vi "TTL high.vi"(1 "Line":i32, 2 "Port":i32, 3 "Do this?":bool=TRUE, 4 "Input":i64[][](array[numeric])=[[-64400000, 1, 6, 0], [-64399000, 0, 12, 0], [-64398000, 0, 12, 1], [-900000, 1, 9, 1], [0, 0, 4, 0], [0, 0, 9, 1], [0, 0, 15, 1], [0, 1, 0, 1], [0, 1, 1, 1], [0, 1, 2, 0], [0, 1, 3, 0], [0, 1, 4, 0], [0, 1, 5, 1], [0, 1, 12, 1], [1000, 1, 7, 0], [10000, 0, 2, 0], [495000, 0, 10, 1], [499000, 0, 6, 0], [501000, 0, 6, 1], [520000, 0, 10, 0], [869000, 0, 11, 1], [896000, 0, 2, 0], [896500, 0, 3, 1], [896500, 0, 9, 0], [896500, 0, 13, 0], [897000, 0, 5, 0], [897000, 1, 7, 1], [898740, 1, 12, 0], [899000, 0, 1, 1], [899000, 0, 4, 0], [899000, 0, 11, 0], [899000, 1, 1, 0], [899000, 1, 13, 1], [899200, 0, 14, 0], [899350, 0, 2, 0], [899400, 0, 14, 1], [899500, 0, 1, 0], [899500, 0, 2, 0], [899500, 0, 4, 0], [900000, 0, 2, 0], [900000, 0, 13, 0], [900000, 1, 1, 1], [900000, 1, 4, 1], [900000, 1, 5, 0], [900000, 1, 7, 0], [900000, 1, 12, 1], [901000, 0, 3, 0], [904000, 0, 5, 0], [904000, 1, 13, 0]], 5 "Absolute start time (ms)":dbl=1400.0 format="%.3f") -> (0 "Output":i64[][](array[numeric])=[[-64400000, 1, 6, 0], [-64399000, 0, 12, 0], [-64398000, 0, 12, 1], [-900000, 1, 9, 1], [0, 0, 4, 0], [0, 0, 9, 1], [0, 0, 15, 1], [0, 1, 0, 1], [0, 1, 1, 1], [0, 1, 2, 0], [0, 1, 3, 0], [0, 1, 4, 0], [0, 1, 5, 1], [0, 1, 12, 1], [1000, 1, 7, 0], [10000, 0, 2, 0], [495000, 0, 10, 1], [499000, 0, 6, 0], [501000, 0, 6, 1], [520000, 0, 10, 0], [869000, 0, 11, 1], [896000, 0, 2, 0], [896500, 0, 3, 1], [896500, 0, 9, 0], [896500, 0, 13, 0], [897000, 0, 5, 0], [897000, 1, 7, 1], [898740, 1, 12, 0], [899000, 0, 1, 1], [899000, 0, 4, 0], [899000, 0, 11, 0], [899000, 1, 1, 0], [899000, 1, 13, 1], [899200, 0, 14, 0], [899350, 0, 2, 0], [899400, 0, 14, 1], [899500, 0, 1, 0], [899500, 0, 2, 0], [899500, 0, 4, 0], [900000, 0, 2, 0], [900000, 0, 13, 0], [900000, 1, 1, 1], [900000, 1, 4, 1], [900000, 1, 5, 0], [900000, 1, 7, 0], [900000, 1, 12, 1], [901000, 0, 3, 0], [904000, 0, 5, 0], [904000, 1, 13, 0], [1398000, 0, 9, 1], [1398000, 0, 15, 1], [1398000, 1, 0, 1], [1400000, 0, 4, 0], [1400000, 1, 1, 1], [1400000, 1, 2, 0], [1400000, 1, 3, 0], [1400000, 1, 4, 0], [1400000, 1, 5, 1], [1400000, 1, 12, 1], [1401000, 1, 7, 0]])   [LabVIEW 2017]
doc: "This subVI turns a single TTL high. Inputs are an input array, time, enable, and two parameter (port and line). Output is an output array = input array plus single TTL high event. Port 1-4 means A-D."
uses:
  globals/DIO board parameters global.vi
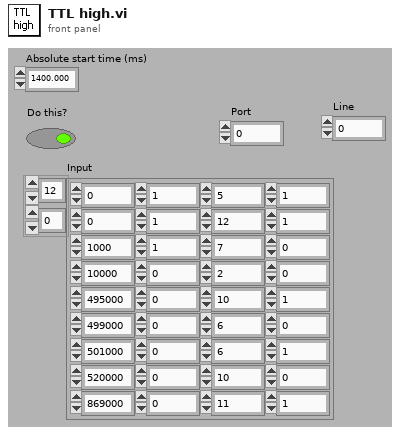
[diagram p1: front panel]
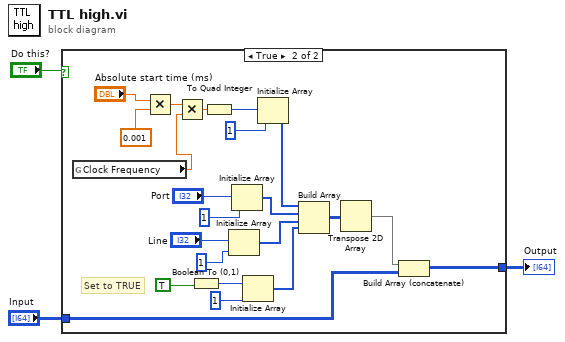
[diagram p0: block diagram]
diagram:
  n1 = case shown="True" "Do this?" {
    tunnel: [w4 w8] -> w2
    tunnel: "Input" -> [w4 w17]
    frame False {
    }
    frame True {
      # "Set to TRUE"
      n2 = global read "DIO board parameters global.vi" "Clock Frequency"() -> (w7:dbl)
      n3 = Multiply(x="Absolute start time (ms)", y=0.001) -> (x*y=w25:dbl)
      n4 = Multiply(x=w25, y=w7) -> (x*y=w6:dbl)
      n5 = Boolean To (0,1)(Boolean=TRUE) -> (0, 1=w20:i16)
      n6 = To Quad Integer(1:w6) -> (0:w5:i64)
      n7 = Initialize Array("Line", 1) -> (w9:i32[])
      n8 = Initialize Array("Port", 1) -> (w10:i32[])
      n9 = Initialize Array(w20, 1) -> (w18:i16[])
      n10 = Initialize Array(w5, 1) -> (w22:i64[])
      n11 = Build Array(w22, w10, w9, w18) -> (w16:i64[][])
      n12 = Transpose 2D Array(2D array=w16) -> (transposed array=w15:i64[][])
      n13 = Build Array (concatenate)(w15, w17) -> (w8:i64[][])
    }
  }
  "Output" <- w2
